vi "add2.vi"() -> ()   [LabVIEW 2020]
panel:
  out "error out":errorcluster caption="错误输出"
  out "a+b":dbl
  in  "b":dbl
  in  "a":dbl
  in  "路径":path
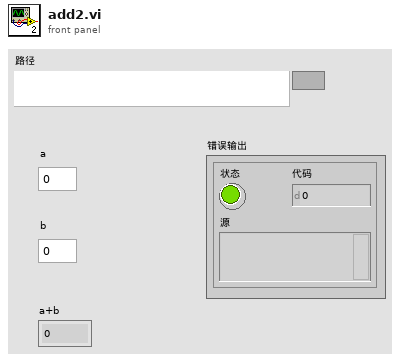
[diagram p1: front panel]
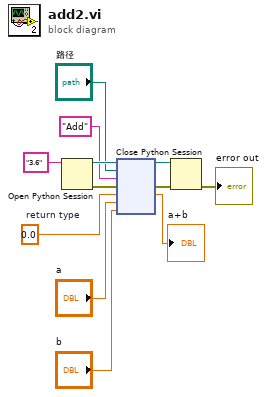
[diagram p0: block diagram]
diagram:
  w7 = 0.0  # return type
  n1 = Open Python Session(python version="3.6") -> (session out=w11:refnum<k35>, error out=w3:errorcluster)  [unwired: 2 in]
  n2 = node(w11, "路径", "Add", w3, w7, "a", "b") -> (w10:refnum<k35>, w2:errorcluster, →"a+b":dbl)  [unwired: 2 in, 2 out]
  n3 = Close Python Session(session in=w10, error in=w2) -> (11:→"error out":errorcluster)
